vi "BarcodeprintR567B.vi"(0 "二维图片 2":picture, 1 "字符串":string) -> (2 "图号":string, 3 "法规号":string)   [LabVIEW 2020]
uses:
  Sources/Global_Variable/Global.vi
panel:
  # "S"
  # "SW  VER: 00.01.00\nHW  VER: 0.0.1"
  # "201ABL\n4BS"
  # "CHN"
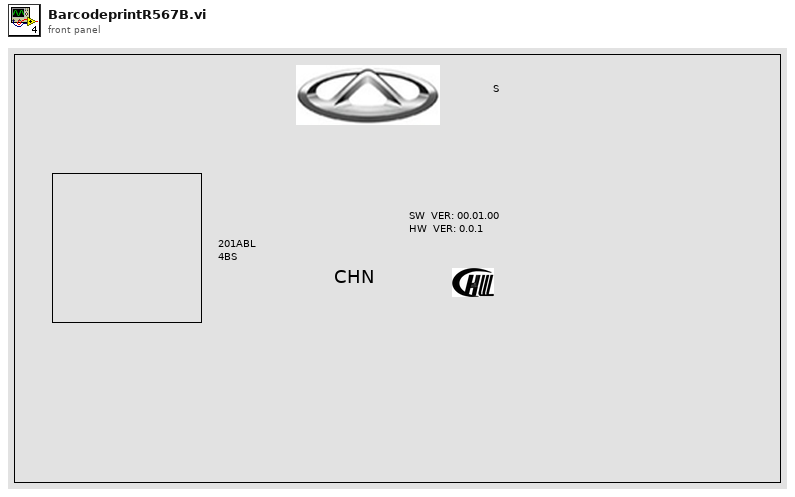
[diagram p1: front panel]
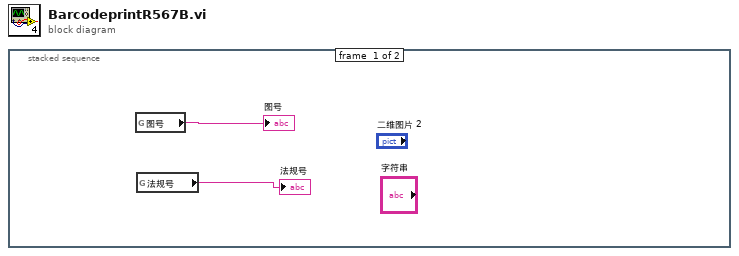
[diagram p0: block diagram]
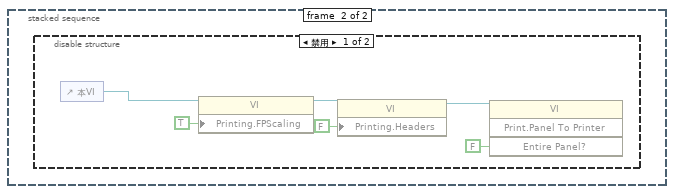
[diagram p2: hidden frame]
diagram:
  n1 = stacked-sequence {
    frame #0 {
      n2 = global read "Global.vi" "图号"() -> (→"图号":string)
      n3 = global read "Global.vi" "法规号"() -> (→"法规号":string)
    }
    frame #1 {
      n4 = disable-structure shown="禁用" {
        frame Disabled {
          n5 = control-ref of="本VI"() -> (w8:refnum<vi>)
          n6 = property class="VI"(reference=w8, "Printing.FPScaling"=TRUE ("打印:前面板缩放？")) -> (reference out=w6:refnum<vi>)  [unwired: 1 in, 1 out]
          n7 = property class="VI"(reference=w6, "Printing.Headers"=FALSE ("打印:页眉？")) -> (reference out=w4:refnum<vi>)  [unwired: 1 in, 1 out]
          n8 = invoke class="VI" method="Print.Panel To Printer"(reference=w4, "Entire Panel?"=FALSE ("整个前面板？")) -> ()  [unwired: 2 in, 4 out]
        }
        frame Enabled {
        }
      }
    }
  }
